vi "Power graph.vi"() -> ()   [LabVIEW 2020]
uses:
  <vilib>/Analysis/2dsp.llb/Integral Method.ctl
  <vilib>/Analysis/8numeric.llb/1D Numeric Integration.vi
  <vilib>/Utility/file.llb/Read Delimited Spreadsheet (DBL).vi
  <vilib>/Analysis/NI_AALPro.lvlib
panel:
  out "result":dbl format="%0.4f"
  out "sum 2":dbl
  out "Integral X 2":dbl[](array[numeric])
  out "Our MFC Power graph 4":dbl[](graph)
  out "all rows":dbl[][](array[numeric])
  in  "file path (dialog if empty)":path=path "C:/Users/boobo/Desktop/19 jan edited.csv"
  out "sum":dbl
  out "Integral X":dbl[](array[numeric])
  out "Our MFC Power graph 3":dbl[](graph)
  out "all rows 2":dbl[][](array[numeric])
  in  "file path (dialog if empty) 3":path=path "C:/Users/boobo/Desktop/FYP labview/data points/200 Data points.csv"
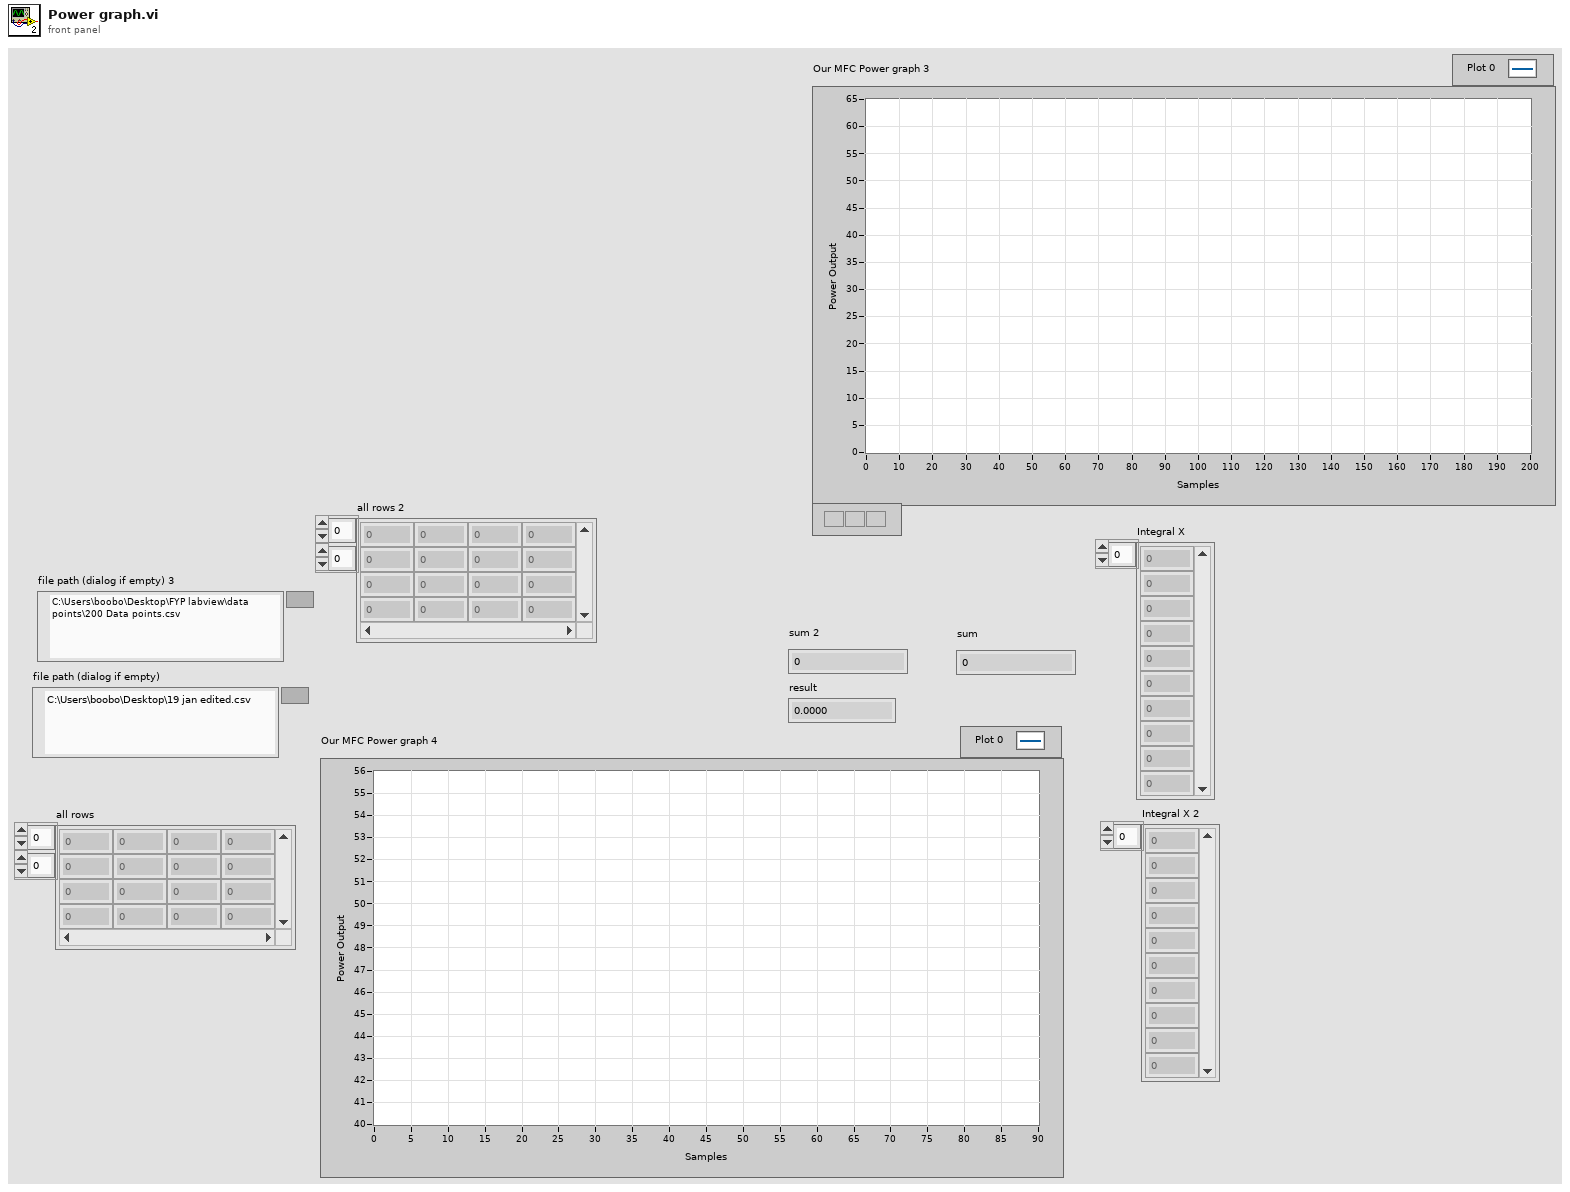
[diagram p1: front panel]
types:
  T1 = typedef "NI_AALPro.lvlib/Integral Method.ctl" = i32
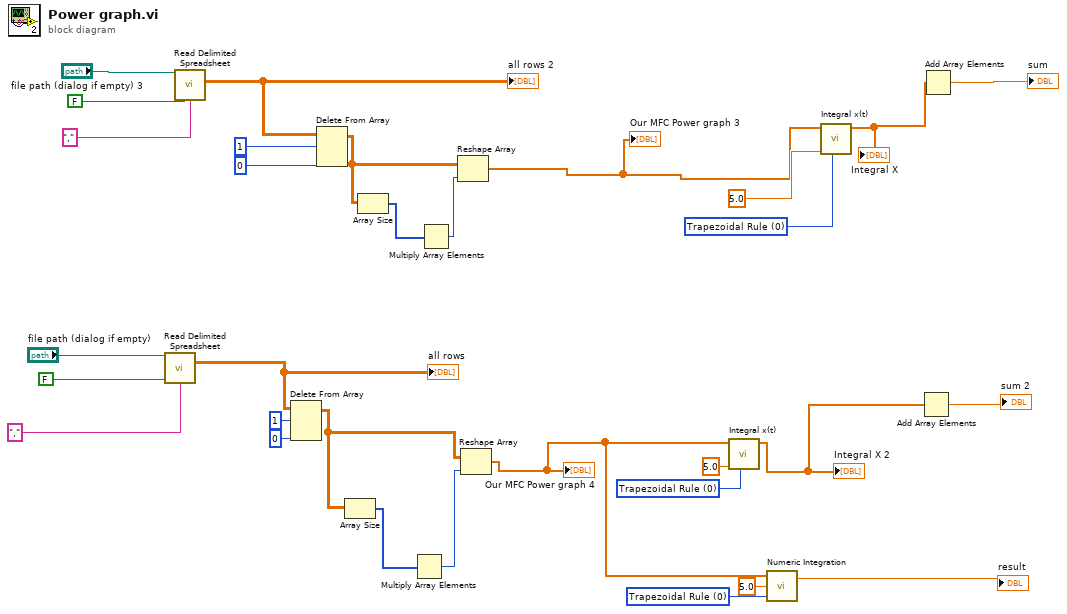
[diagram p0: block diagram]
diagram:
  w4 = T1 0 items=["Trapezoidal Rule", "Simpson's Rule", "Simpson's 3/8 Rule", "Bode Rule"] ("integration method")
  w7 = T1 0 items=["Trapezoidal Rule", "Simpson's Rule", "Simpson's 3/8 Rule", "Bode Rule"] ("integration method")
  w22 = T1 0 items=["Trapezoidal Rule", "Simpson's Rule", "Simpson's 3/8 Rule", "Bode Rule"] ("integration method")
  n1 = call-poly <vilib>:"Read Delimited Spreadsheet.vi"("file path (dialog if empty)"="file path (dialog if empty)", "transpose? (F)"=FALSE, "delimiter (\\t)"="," ("delimiter (\\t)")) -> ("all rows"=w15:dbl[][])  [unwired: 7 in, 5 out]
  "all rows" <- w15
  n2 = call-poly <vilib>:"Read Delimited Spreadsheet.vi"("file path (dialog if empty)"="file path (dialog if empty) 3", "transpose? (F)"=FALSE, "delimiter (\\t)"="," ("delimiter (\\t)")) -> ("all rows"=w28:dbl[][])  [unwired: 7 in, 5 out]
  "all rows 2" <- w28
  n3 = Delete From Array "Delete From Array"(array=w15, length=1, index (row)=0) -> (array with subset deleted=w12:dbl[][])  [unwired: 1 in, 1 out]
  n4 = Delete From Array "Delete From Array"(array=w28, length=1, index (row)=0) -> (array with subset deleted=w23:dbl[][])  [unwired: 1 in, 1 out]
  n5 = Array Size(array=w12) -> (size(s)=w11:i32[])
  n6 = Array Size(array=w23) -> (size(s)=w25:i32[])
  n7 = Multiply Array Elements(1:w11) -> (0:w10:i32)
  n8 = Multiply Array Elements(1:w25) -> (0:w24:i32)
  n9 = Reshape Array "Reshape Array"(w23, w24) -> (w5:dbl[])
  "Our MFC Power graph 3" <- w5
  n10 = Reshape Array "Reshape Array"(w12, w10) -> (w3:dbl[])
  "Our MFC Power graph 4" <- w3
  n11 = call <vilib>:"Integral x(t).vi"("integration method"=w7, "dt"=5.0, "X"=w3) -> ("Integral X"=w6:dbl[])  [unwired: 7 in, 1 out]
  "Integral X 2" <- w6
  n12 = call-poly <vilib>:"Numeric Integration.vi"("integration method"=w4, "dt"=5.0, "Input Array"=w3) -> ("result"=→"result":dbl)  [unwired: 1 out]
  n13 = call <vilib>:"Integral x(t).vi"("integration method"=w22, "dt"=5.0, "X"=w5) -> ("Integral X"=w21:dbl[])  [unwired: 7 in, 1 out]
  "Integral X" <- w21
  n14 = Add Array Elements(numeric array=w6) -> (sum=→"sum 2":dbl)
  n15 = Add Array Elements(numeric array=w21) -> (sum=→"sum":dbl)
